vi "Polygon Area.vi"(10 "Y":dbl[](array[numeric]), 11 "X":dbl[](array[numeric])) -> (0 "error":i32, 3 "signed area":dbl)   [LabVIEW 2020, in "NI_AAL_Geometry.lvlib"]
doc: "Calculates the signed area of a simple polygon."
uses:
  <vilib>/Analysis/NI_AAL_Geometry.lvlib
  <vilib>/Analysis/baseanly.llb/Real Dot Product.vi
  <vilib>/Analysis/NI_AALBase.lvlib
panel:
  # "Polygon Area"
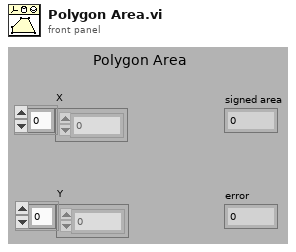
[diagram p1: front panel]
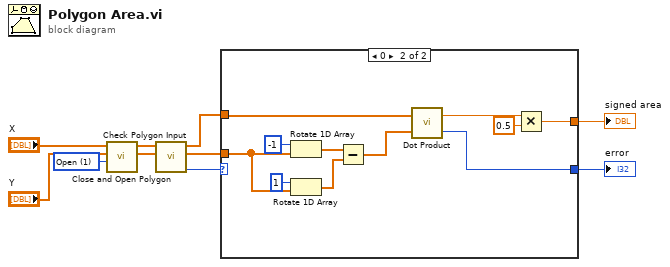
[diagram p0: block diagram]
diagram:
  w7 = u16 1 items=["Closed", "Open"] ("type")
  n1 = call <vilib>:"Close and Open Polygon.vi"("type"=w7, "Y In"="Y", "X In"="X") -> ("Y Out"=w5:dbl[], "X Out"=w6:dbl[])  [unwired: 7 in]
  n2 = call <vilib>:"Check Polygon Input.vi"("Y In"=w5, "X In"=w6) -> ("error"=w8:i32, "Y Out"=w10:dbl[], "X Out"=w9:dbl[])  [unwired: 7 in]
  n3 = case shown="0" w8 {
    selector: w8 -> [w11 _]
    tunnel: [_ w12] -> w2
    tunnel: w9 -> [_ w15]
    tunnel: w10 -> [_ w14]
    tunnel: [w11 w13] -> w1
    frame -1, Default {
    }
    frame 0 {
      n4 = Rotate 1D Array(1:w14, 2:-1 ("n")) -> (0:w16:dbl[])
      n5 = Rotate 1D Array(1:w14, 2:1 ("n")) -> (0:w20:dbl[])
      n6 = Subtract(x=w16, y=w20) -> (x-y=w19:dbl[])
      n7 = call-poly <vilib>:"Dot Product.vi"("Y Vector"=w19, "X Vector"=w15) -> ("error"=w13:i32, "X * Y"=w18:dbl)
      n8 = Multiply(x=w18, y=0.5) -> (x*y=w12:dbl)
    }
  }
  "signed area" <- w2
  "error" <- w1
